vi "oa_AC DC Separation Exp (N Channel).vi"(7 "reset? (F)":bool, 8 "points/rev":u32, 9 "averaging revolution (1)":dbl=1.0 min=0.0, 11 "even angle signals":cluster{"r0":dbl, "dr":dbl, "Y":dbl[]}[](array[cluster]) {"r0" format="%.2p"; "dr" format="%.2p"; "Y" format="%.2f"}) -> (0 "DC even angle signals":cluster{"r0":dbl, "dr":dbl, "Y":dbl[]}[](array[cluster]), 1 "AC even angle signals":cluster{"r0":dbl, "dr":dbl, "Y":dbl[]}[](array[cluster]), 3 "dul even angle signals":cluster{"r0":dbl, "dr":dbl, "Y":dbl[]}[](array[cluster]))   [LabVIEW 2017, in "SoundVib_OAUtility.lvlib"]
uses:
  <vilib>/addons/Sound and Vibration/Order Analysis/Utility/SoundVib_OAUtility.lvlib
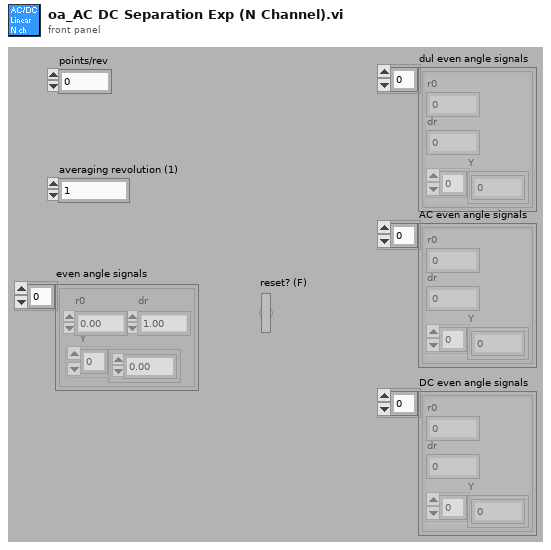
[diagram p1: front panel]
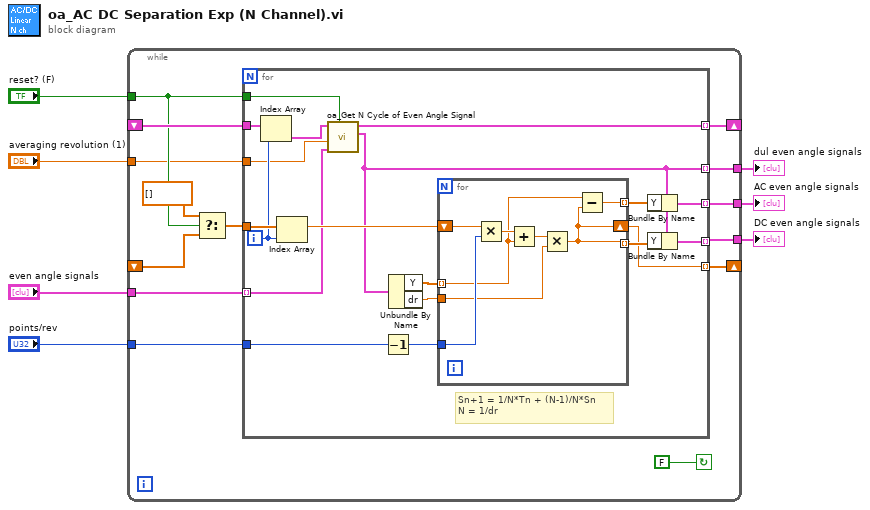
[diagram p0: block diagram]
diagram:
  n1 = while {
    tunnel: "even angle signals" -> [w19]
    tunnel: "reset? (F)" -> [w10]
    shift-right: [w17] -> _
    shift-left: _ -> [w20]
    tunnel: [w16] -> w3
    tunnel: [w15] -> w2
    tunnel: "points/rev" -> [w14]
    shift-right: [w11] -> _
    shift-left: _ -> [w12]
    tunnel: [w9] -> w4
    tunnel: "averaging revolution (1)" -> [w8]
    stop <- FALSE continue-if-true
    n2 = Select(t=dbl[] [], s=w10, f=w20) -> (s? t:f=w18:dbl[])
    n3 = for {
      tunnel: w19 -> [w29] mode=indexing
      tunnel: w18 -> [w40]
      tunnel: [w33] -> w17 mode=indexing
      tunnel: [w32] -> w16 mode=indexing
      tunnel: [w31] -> w15 mode=indexing
      tunnel: w14 -> [w30]
      tunnel: w12 -> [w25]
      tunnel: [w26] -> w11 mode=indexing
      tunnel: w10 -> [w24]
      tunnel: [w23] -> w9 mode=indexing
      tunnel: w8 -> [w22]
      i -> [w28]
      # "Sn+1 = 1/N*Tn + (N-1)/N*Sn\nN = 1/dr"
      n4 = Index Array(array=w25, index=w28) -> (element=w27:cluster{"r0":dbl, "dr":dbl, "Y":dbl[]})
      n5 = Index Array(array=w40, index=w28) -> (element=w34:dbl)
      n6 = call <vilib>:"oa_Get N Cycle of Even Angle Signal.vi"("reset"=w24, "new even angle signal"=w29, "averaging revolution (1)"=w22, "rest even angle signal"=w27) -> ("even angle signal"=w23:cluster{"r0":dbl, "dr":dbl, "Y":dbl[]}, "rest even angle signal out"=w26:cluster{"r0":dbl, "dr":dbl, "Y":dbl[]})  [unwired: 4 in, 2 out]
      n7 = Decrement(x=w30) -> (x-1=w36:u32)
      n8 = Unbundle By Name(w23) -> ("Y"=w35:dbl[], "dr"=w37:dbl)
      n9 = for {
        shift-right: [w41] -> w33
        shift-left: w34 -> [w48]
        tunnel: w35 -> [w43] mode=indexing
        tunnel: w36 -> [w45]
        tunnel: w37 -> [w44]
        tunnel: [w42] -> w38 mode=indexing
        tunnel: [w41] -> w39 mode=indexing
        n10 = Multiply(x=w48, y=w45) -> (x*y=w47:dbl)
        n11 = Add(x=w47, y=w43) -> (x+y=w46:dbl)
        n12 = Multiply(x=w46, y=w44) -> (x*y=w41:dbl)
        n13 = Subtract(x=w43, y=w41) -> (x-y=w42:dbl)
      }
      n14 = Bundle By Name(cluster=w23, "Y"=w38) -> (w32:cluster{"r0":dbl, "dr":dbl, "Y":dbl[]})
      n15 = Bundle By Name(cluster=w23, "Y"=w39) -> (w31:cluster{"r0":dbl, "dr":dbl, "Y":dbl[]})
    }
  }
  "dul even angle signals" <- w4
  "AC even angle signals" <- w3
  "DC even angle signals" <- w2
